vi "Autonomous Independent.vi"() -> ()   [LabVIEW 2014]
doc: "This VI is called when autonomous begins, and will automatically be terminated when autonomous ends. You can carry out timed or sensor driven robot movement independently without needing to return to the caller."
uses:
  <vilib>/Rock Robotics/WPI/Solenoid/WPI_SolenoidValue.ctl
  Robot Global Data.vi
  <vilib>/Rock Robotics/WPI/RobotDrive/WPI_RobotDriveGetSetRefNum.vi
  <vilib>/Rock Robotics/WPI/Solenoid/WPI_SolenoidSetEnum.vi
panel:
  out "One Ball Timer 1":u32
  out "Timer 2":u32
  out "Timer 1":u32
  out "Both Hands In":i32
  out "Av. Goalie 1 Ball Timer":u32
  out "Anti-Defense Iterations":dbl
  out "auton mode selected":string
  in  "pickup arm gripping speed":dbl=0.3
  in  "Speed Control":dbl=-0.46
  # "Be sure to right-click and choose Data Operations>>Make Current Value default if you want to save the array values with the VI"
  # "-0.46 < -0.48 <-0.51 -0.55< -0.43 < -0.5 < -0.58\n(Newest < New < Old < Oldest)"
  # "0.3"
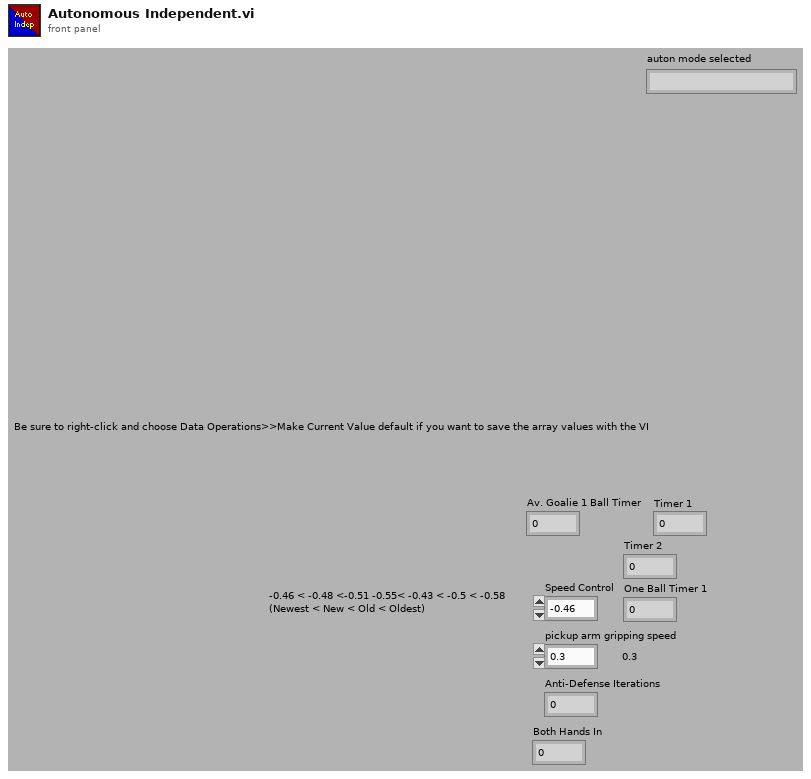
[diagram p1: front panel]
types:
  T1 = typedef "WPI_RobotDriveDevRef.ctl" = cluster{"DevStatus":errorcluster, "Motors[]":T2[], "Square Inputs":bool, "Max Output":dbl}
  T2 = typedef "WPI_MotorControlDeviceRef.ctl" = cluster{"DeviceStatus":errorcluster, "Type":enum16{"PWM", "CAN"}, "PWM":cluster{"Digital Module":T3, "PWM Channel":T4, "DeadBand":T5}, "CAN":cluster{"Device Number":u8, "Control Mode":T6, "Semaphore":T7, "Max Vout":dbl}, "Invert":bool, "TransformRef":T8, "InvTransformRef":T8}
  T3 = typedef "FPGA_TypedefDigitalModule.ctl" = enum16{"Digital Module 1", "Digital Module 2"}
  T4 = typedef "FPGA_DIOPWMChannel.ctl" = enum8{"PWM 1", "PWM 2", "PWM 3", "PWM 4", "PWM 5", "PWM 6", "PWM 7", "PWM 8", "PWM 9", "PWM 10", "Invalid"}
  T5 = typedef "WPI_PWMDeadband.ctl" = cluster{"Name":string, "maxPositivePwm":i32, "minPositivePwm":i32, "centerPwm":i32, "maxNegativePwm":i32, "minNegativePwm":i32, "angularRange":u16}
  T6 = typedef "WPI_CANJaguar_ControlMode.ctl" = enum8{"Percent VBus", "Current", "Speed", "Position", "Voltage"}
  T7 = typedef "Semaphore RefNum" = refnum<k1>
  T8 = typedef "WPI_PWMTransform_ConPane.ctl" = refnum<vi>
  T9 = typedef "WPI_AnalogChannelDevRef.ctl" = cluster{"DevStatus":errorcluster, "Analog Module":T10, "Analog Channel":T11}
  T10 = typedef "FPGA_TypedefAnalogModule.ctl" = enum16{"Analog Module 1", "Analog Module 2"}
  T11 = typedef "FPGA_AIChannel.ctl" = enum8{"AI 1", "AI 2", "AI 3", "AI 4", "AI 5", "AI 6", "AI 7", "AI 8", "Invalid"}
  T12 = typedef "WPI_SolenoidDevRef.ctl" = cluster{"DevStatus":errorcluster, "Solenoid Module":T13, "Forward Solenoid Channel":T14, "Reverse Solenoid Channel":T14}
  T13 = typedef "FPGA_TypedefSolenoidModule.ctl" = enum16{"Solenoid Module 1", "Solenoid Module 2"}
  T14 = typedef "WPI_SolenoidChannel.ctl" = enum8{"Solenoid 1", "Solenoid 2", "Solenoid 3", "Solenoid 4", "Solenoid 5", "Solenoid 6", "Solenoid 7", "Solenoid 8", "Invalid"}
  T15 = typedef "WPI_SolenoidValue.ctl" = enum16{"Off", "On", "Forward", "Reverse"}
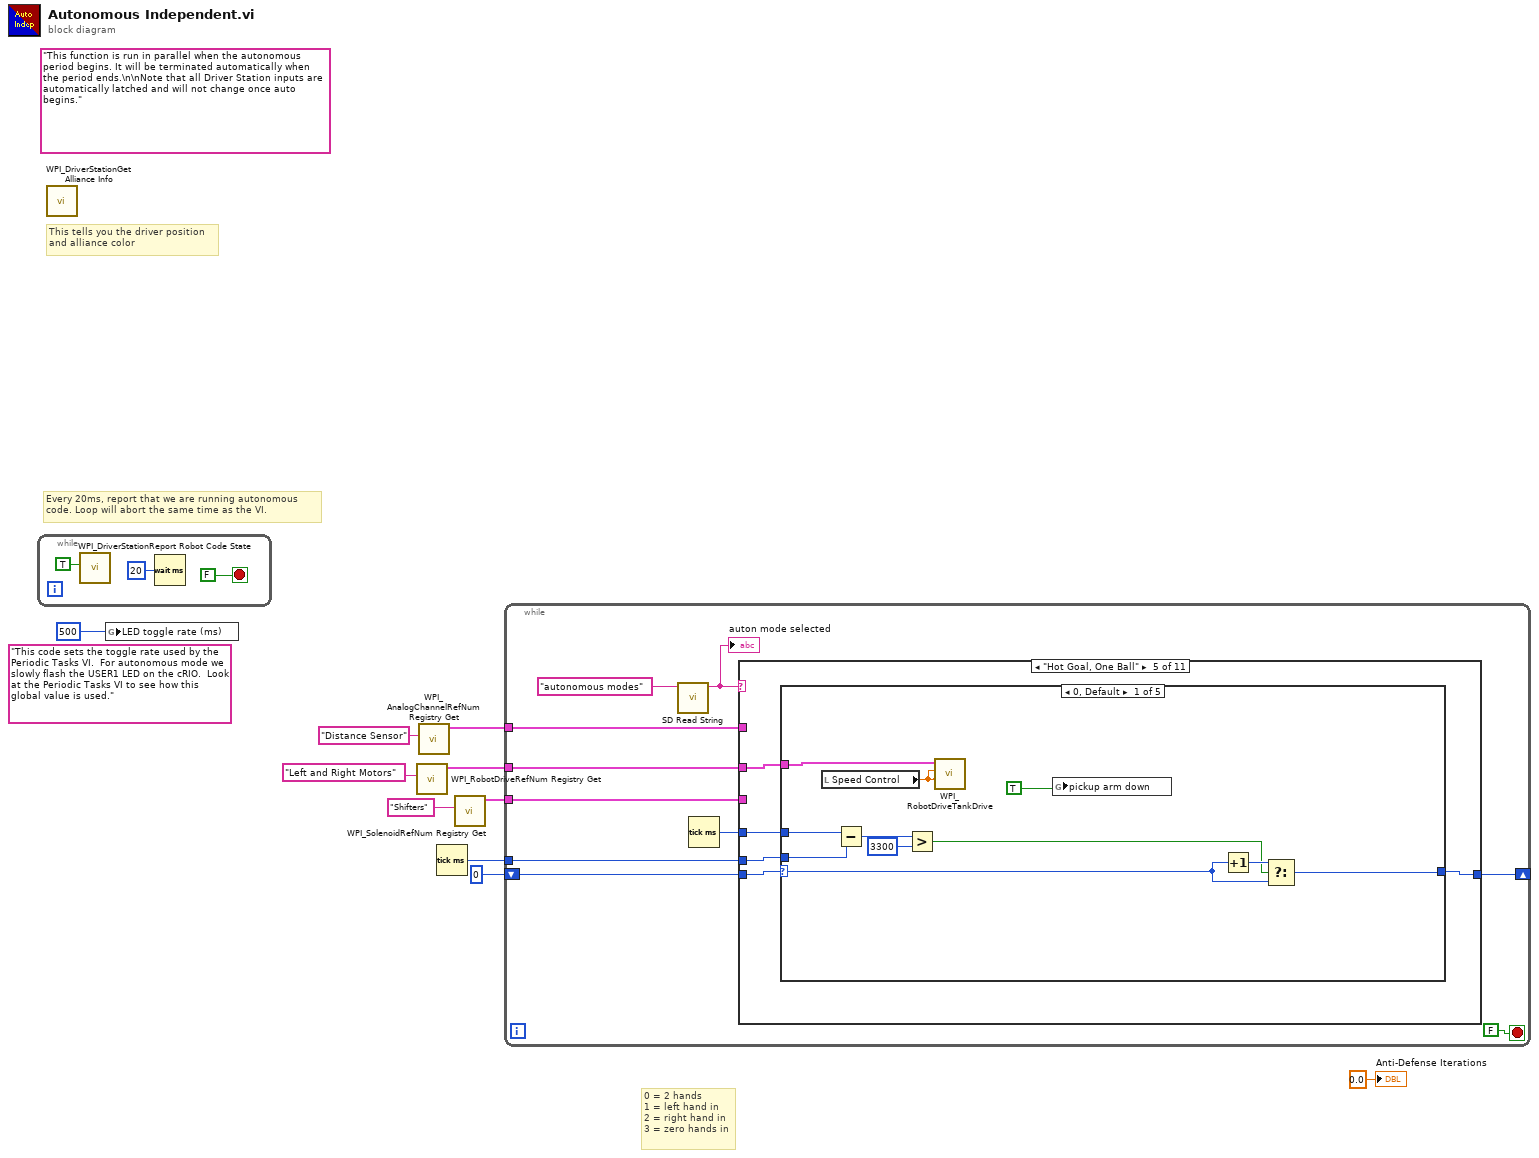
[diagram p0: block diagram]
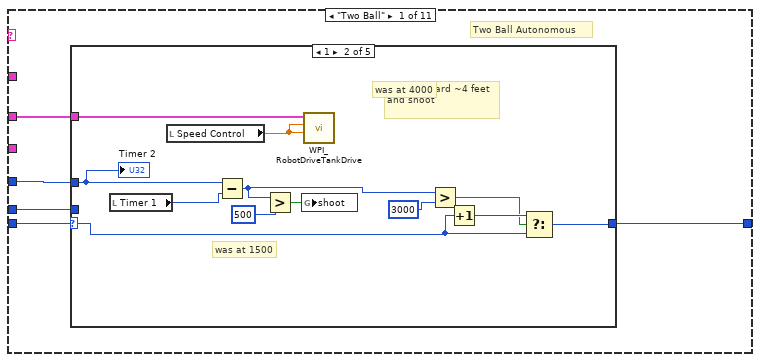
[diagram p2: hidden frame]
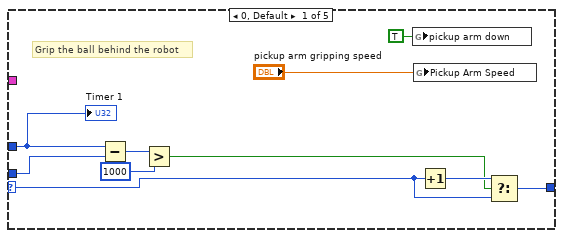
[diagram p3: hidden frame]
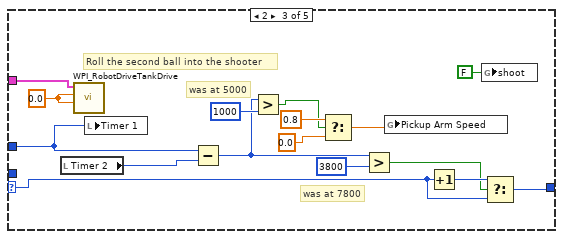
[diagram p4: hidden frame]
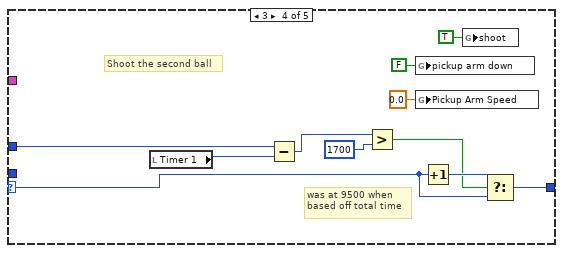
[diagram p5: hidden frame]
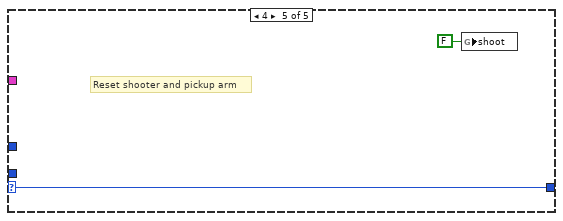
[diagram p6: hidden frame]
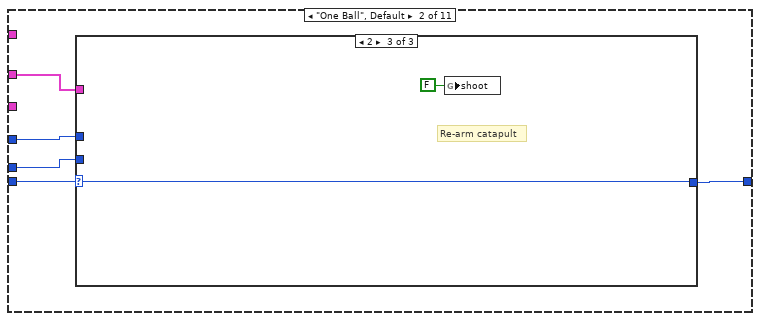
[diagram p7: hidden frame]
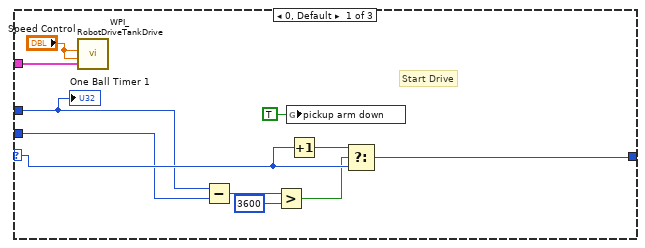
[diagram p8: hidden frame]
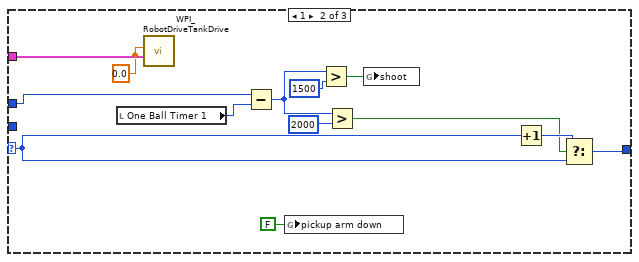
[diagram p9: hidden frame]
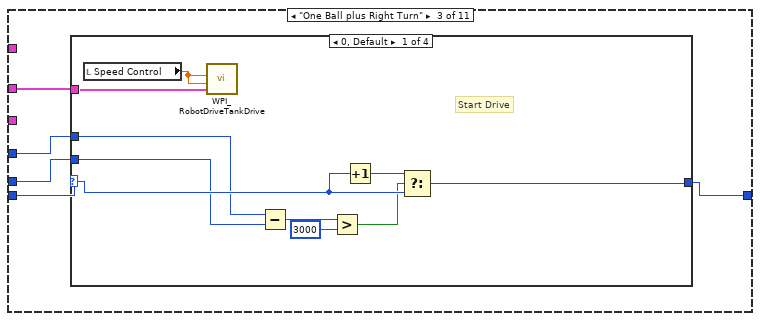
[diagram p10: hidden frame]
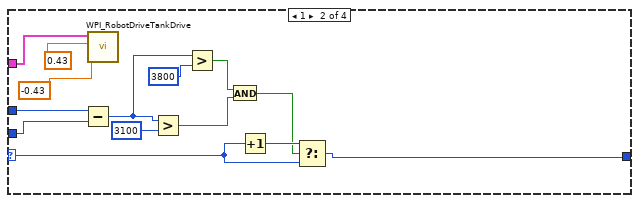
[diagram p11: hidden frame]
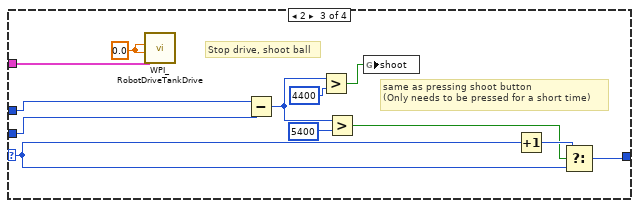
[diagram p12: hidden frame]
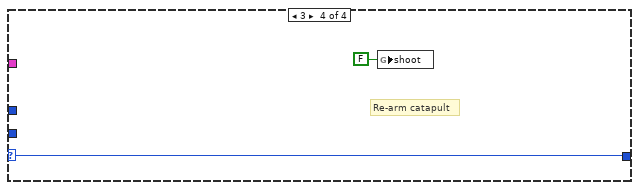
[diagram p13: hidden frame]
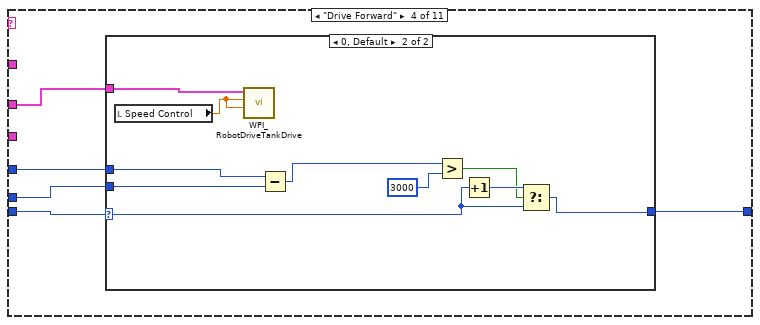
[diagram p14: hidden frame]
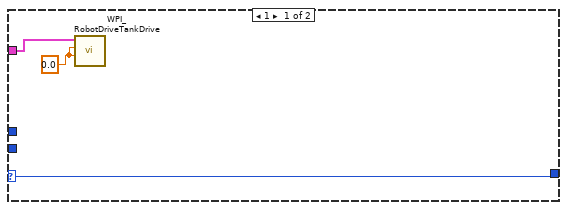
[diagram p15: hidden frame]
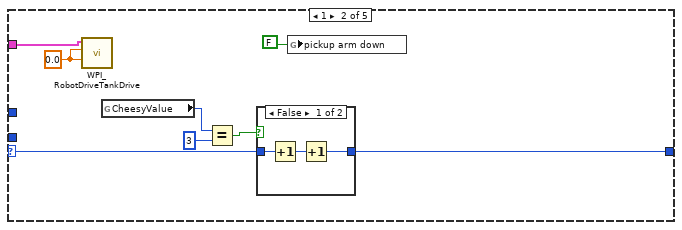
[diagram p16: hidden frame]
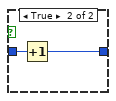
[diagram p17: hidden frame]
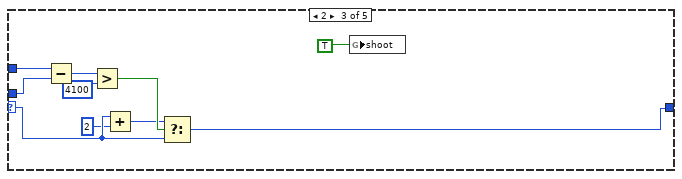
[diagram p18: hidden frame]
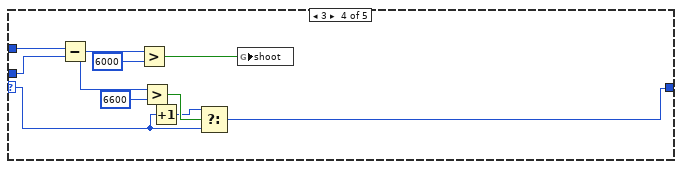
[diagram p19: hidden frame]
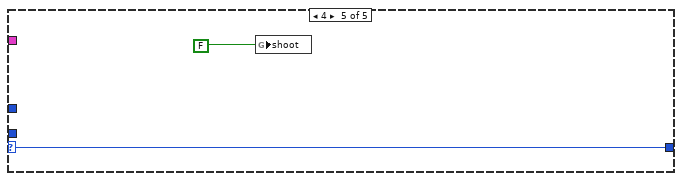
[diagram p20: hidden frame]
diagram:
  (unwired) "This code sets the toggle rate used by the Periodic Tasks VI.  For autonomous mode we slowly flash the USER1 LED on the cRIO.  Look at the Periodic Tasks VI to see how this global value is used."
  (unwired) "This function is run in parallel when the autonomous period begins. It will be terminated automatically when the period ends.\n\nNote that all Driver Station inputs are automatically latched and will not change once auto begins."
  # "0 = 2 hands\n1 = left hand in\n2 = right hand in\n3 = zero hands in"
  # "Every 20ms, report that we are running autonomous\ncode. Loop will abort the same time as the VI."
  # "This tells you the driver position\nand alliance color"
  n1 = while {
    stop <- FALSE stop-if-true
    n2 = call <vilib>:"WPI_DriverStationReport Robot Code State.vi"("Autonomous"=TRUE) -> ()  [unwired: 10 in, 1 out]
    n3 = Wait (ms)(milliseconds to wait=u32 20) -> ()  [unwired: 1 out]
  }
  n4 = call <vilib>:"WPI_DriverStationGet Alliance Info.vi"() -> ()  [unwired: 12 out]
  n5 = global write "Robot Global Data.vi" "LED toggle rate (ms)"(u32 500 ("LED ms toggle rate")) -> ()
  n6 = call <vilib>:"WPI_RobotDriveRefNum Registry Get.vi"("refnum name"="Left and Right Motors") -> ("RobotDriveDevRef"=w7:T1)  [unwired: 9 in, 1 out]
  n7 = call <vilib>:"WPI_AnalogChannelRefNum Registry Get.vi"("refnum name"="Distance Sensor") -> ("AIDeviceRef"=w1:T9)  [unwired: 9 in, 1 out]
  n8 = Tick Count (ms)() -> (millisecond timer value=w9:u32)
  n9 = call <vilib>:"WPI_SolenoidRefNum Registry Get.vi"("refnum name"="Shifters") -> ("SolenoidDevRef"=w4:T12)  [unwired: 9 in, 1 out]
  n10 = while {
    shift-right: [w19] -> _
    shift-left: 0 -> [w22]
    tunnel: w9 -> [w20]
    tunnel: w7 -> [w16]
    tunnel: w4 -> [w15]
    tunnel: w1 -> [w14]
    stop <- FALSE stop-if-true
    n11 = call <vilib>:"SD Read String.vi"("Name"="autonomous modes") -> ("String"=w17:string)  [unwired: 8 in, 2 out]
    "auton mode selected" <- w17
    n12 = Tick Count (ms)() -> (millisecond timer value=w21:u32)
    n13 = case shown="\"Hot Goal, One Ball\"" w17 {
      tunnel: w22 -> [w28 w83 w115 w155 w175 w227 w260 w308 w360 w472 w509]
      tunnel: w21 -> [w27 w82 w113 w157 w174 w223 w256 w307 w359 _ w508]
      tunnel: w20 -> [w26 w81 w114 w156 w173 _ _ w306 w358 _ w507]
      tunnel: [w25 w80 w111 w154 w176 w224 w257 w309 w357 w472 w506] -> w19
      tunnel: w16 -> [w24 w84 w112 w158 w172 w226 w259 w305 w361 w470 w505]
      tunnel: w15 -> [_ _ _ _ _ _ _ _ _ w469 _]
      tunnel: w14 -> [_ _ _ _ _ w228 w261 _ _ _ _]
      frame "Two Ball" {
        # "Two Ball Autonomous"
        n14 = case shown="1" w28 {
          selector: w28 -> [w30 w42 w65 w75 w79]
          tunnel: w27 -> [w29 w44 w52 w72 _]
          tunnel: w26 -> [w36 _ _ _ _]
          tunnel: [w33 w47 w62 w74 w79] -> w25
          tunnel: w24 -> [_ w50 w59 _ _]
          frame 0, Default {
            # "Grip the ball behind the robot"
            n15 = Subtract(x=w29, y=w36) -> (x-y=w35:u32)
            n16 = Greater?(x=w35, y=u32 1000) -> (0:w31:bool)
            n17 = global write "Robot Global Data.vi" "pickup arm down"(TRUE ("pickup arm down")) -> ()
            n18 = global write "Robot Global Data.vi" "Pickup Arm Speed"("pickup arm gripping speed") -> ()
            n19 = Increment(x=w30) -> (x+1=w32:u32)
            n20 = Select(t=w32, s=w31, f=w30) -> (s? t:f=w33:u32)
            "Timer 1" <- w29
          }
          frame 1 {
            # "was at 4000"
            # "was at 1500"
            # "Drive forward ~4 feet and shoot"
            n21 = local read "Timer 1"() -> (w39:u32)
            n22 = local read "Speed Control"() -> (w40:dbl)
            n23 = Subtract(x=w44, y=w39) -> (x-y=w46:u32)
            n24 = Greater?(x=w46, y=u32 500) -> (0:w41:bool)
            n25 = global write "Robot Global Data.vi" "shoot"(w41) -> ()
            n26 = call <vilib>:"WPI_RobotDriveTankDrive.vi"("Right axis value"=w40, "Left axis value"=w40, "RobotDriveDevRef"=w50) -> ()  [unwired: 6 in, 3 out]
            n27 = Greater?(x=w46, y=u32 3000) -> (0:w43:bool)
            n28 = Increment(x=w42) -> (x+1=w48:u32)
            n29 = Select(t=w48, s=w43, f=w42) -> (s? t:f=w47:u32)
            "Timer 2" <- w44
          }
          frame 2 {
            w60 = 0.0 ("Left axis value")
            # "was at 7800"
            # "was at 5000"
            # "Roll the second ball into the shooter"
            n30 = local read "Timer 2"() -> (w51:u32)
            n31 = call <vilib>:"WPI_RobotDriveTankDrive.vi"("Right axis value"=w60, "Left axis value"=w60, "RobotDriveDevRef"=w59) -> ()  [unwired: 6 in, 3 out]
            n32 = local write "Timer 1"(w52) -> ()
            n33 = Subtract(x=w52, y=w51) -> (x-y=w54:u32)
            n34 = Greater?(x=w54, y=u32 1000) -> (0:w53:bool)
            n35 = Select(t=0.8 ("Pickup Arm Speed"), s=w53, f=0.0) -> (s? t:f=w56:dbl)
            n36 = Greater?(x=w54, y=u32 3800) -> (0:w63:bool)
            n37 = global write "Robot Global Data.vi" "Pickup Arm Speed"(w56) -> ()
            n38 = Increment(x=w65) -> (x+1=w66:u32)
            n39 = global write "Robot Global Data.vi" "shoot"(FALSE ("shoot")) -> ()
            n40 = Select(t=w66, s=w63, f=w65) -> (s? t:f=w62:u32)
          }
          frame 3 {
            # "was at 9500 when\nbased off total time"
            # "Shoot the second ball"
            n41 = local read "Timer 1"() -> (w67:u32)
            n42 = Subtract(x=w72, y=w67) -> (x-y=w71:u32)
            n43 = Greater?(x=w71, y=u32 1700) -> (0:w69:bool)
            n44 = global write "Robot Global Data.vi" "pickup arm down"(FALSE ("pickup arm down")) -> ()
            n45 = global write "Robot Global Data.vi" "Pickup Arm Speed"(0.0 ("Pickup Arm Speed")) -> ()
            n46 = Increment(x=w75) -> (x+1=w76:u32)
            n47 = global write "Robot Global Data.vi" "shoot"(TRUE ("shoot")) -> ()
            n48 = Select(t=w76, s=w69, f=w75) -> (s? t:f=w74:u32)
          }
          frame 4 {
            # "Reset shooter and pickup arm"
            n49 = global write "Robot Global Data.vi" "shoot"(FALSE ("shoot")) -> ()
          }
        }
      }
      frame "One Ball", Default {
        n50 = case shown="2" w83 {
          selector: w83 -> [w93 w107 w110]
          tunnel: w84 -> [w95 w104 _]
          tunnel: w82 -> [w92 w102 _]
          tunnel: w81 -> [w91 _ _]
          tunnel: [w87 w105 w110] -> w80
          frame 0, Default {
            # "Start Drive"
            n51 = call <vilib>:"WPI_RobotDriveTankDrive.vi"("Right axis value"="Speed Control", "Left axis value"="Speed Control", "RobotDriveDevRef"=w95) -> ()  [unwired: 6 in, 3 out]
            n52 = Subtract(x=w92, y=w91) -> (x-y=w90:u32)
            n53 = Greater?(x=w90, y=u32 3600) -> (0:w88:bool)
            n54 = global write "Robot Global Data.vi" "pickup arm down"(TRUE ("pickup arm down")) -> ()
            n55 = Increment(x=w93) -> (x+1=w94:u32)
            n56 = Select(t=w94, s=w88, f=w93) -> (s? t:f=w87:u32)
            "One Ball Timer 1" <- w92
          }
          frame 1 {
            w103 = 0.0 ("Left axis value")
            n57 = local read "One Ball Timer 1"() -> (w96:u32)
            n58 = call <vilib>:"WPI_RobotDriveTankDrive.vi"("Right axis value"=w103, "Left axis value"=w103, "RobotDriveDevRef"=w104) -> ()  [unwired: 6 in, 3 out]
            n59 = Subtract(x=w102, y=w96) -> (x-y=w100:u32)
            n60 = global write "Robot Global Data.vi" "pickup arm down"(FALSE ("pickup arm down")) -> ()
            n61 = Greater?(x=w100, y=u32 1500) -> (0:w98:bool)
            n62 = Greater?(x=w100, y=u32 2000) -> (0:w101:bool)
            n63 = global write "Robot Global Data.vi" "shoot"(w98) -> ()
            n64 = Increment(x=w107) -> (x+1=w108:u32)
            n65 = Select(t=w108, s=w101, f=w107) -> (s? t:f=w105:u32)
          }
          frame 2 {
            # "Re-arm catapult"
            n66 = global write "Robot Global Data.vi" "shoot"(FALSE ("shoot")) -> ()
          }
        }
      }
      frame "One Ball plus Right Turn" {
        n67 = case shown="0, Default" w115 {
          selector: w115 -> [w123 w130 w150 w153]
          tunnel: w112 -> [w125 w134 w146 _]
          tunnel: w113 -> [w122 w139 w144 _]
          tunnel: w114 -> [w121 w138 w149 _]
          tunnel: [w117 w126 w147 w153] -> w111
          frame 0, Default {
            # "Start Drive"
            n68 = local read "Speed Control"() -> (w116:dbl)
            n69 = call <vilib>:"WPI_RobotDriveTankDrive.vi"("Right axis value"=w116, "Left axis value"=w116, "RobotDriveDevRef"=w125) -> ()  [unwired: 6 in, 3 out]
            n70 = Subtract(x=w122, y=w121) -> (x-y=w120:u32)
            n71 = Greater?(x=w120, y=u32 3000) -> (0:w118:bool)
            n72 = Increment(x=w123) -> (x+1=w124:u32)
            n73 = Select(t=w124, s=w118, f=w123) -> (s? t:f=w117:u32)
          }
          frame 1 {
            n74 = Subtract(x=w139, y=w138) -> (x-y=w136:u32)
            n75 = call <vilib>:"WPI_RobotDriveTankDrive.vi"("Right axis value"=-0.43, "Left axis value"=0.43, "RobotDriveDevRef"=w134) -> ()  [unwired: 6 in, 3 out]
            n76 = Greater?(x=w136, y=u32 3100) -> (0:w128:bool)
            n77 = Greater?(x=w136, y=u32 3800) -> (0:w129:bool)
            n78 = And(x=w129, y=w128) -> (x .and. y?=w127:bool)
            n79 = Increment(x=w130) -> (x+1=w131:u32)
            n80 = Select(t=w131, s=w127, f=w130) -> (s? t:f=w126:u32)
          }
          frame 2 {
            w145 = 0.0 ("Left axis value")
            # "same as pressing shoot button\n(Only needs to be pressed for a short time)"
            # "Stop drive, shoot ball"
            n81 = call <vilib>:"WPI_RobotDriveTankDrive.vi"("Right axis value"=w145, "Left axis value"=w145, "RobotDriveDevRef"=w146) -> ()  [unwired: 6 in, 3 out]
            n82 = Subtract(x=w144, y=w149) -> (x-y=w142:u32)
            n83 = Greater?(x=w142, y=u32 4400) -> (0:w140:bool)
            n84 = Greater?(x=w142, y=u32 5400) -> (0:w143:bool)
            n85 = global write "Robot Global Data.vi" "shoot"(w140) -> ()
            n86 = Increment(x=w150) -> (x+1=w151:u32)
            n87 = Select(t=w151, s=w143, f=w150) -> (s? t:f=w147:u32)
          }
          frame 3 {
            # "Re-arm catapult"
            n88 = global write "Robot Global Data.vi" "shoot"(FALSE ("shoot")) -> ()
          }
        }
      }
      frame "Drive Forward" {
        n89 = case shown="0, Default" w155 {
          selector: w155 -> [w159 w165]
          tunnel: w158 -> [w161 w169]
          tunnel: w157 -> [_ w171]
          tunnel: w156 -> [_ w170]
          tunnel: [w159 w164] -> w154
          frame 1 {
            w160 = 0.0 ("Right axis value")
            n90 = call <vilib>:"WPI_RobotDriveTankDrive.vi"("Right axis value"=w160, "Left axis value"=w160, "RobotDriveDevRef"=w161) -> ()  [unwired: 6 in, 3 out]
          }
          frame 0, Default {
            n91 = local read "Speed Control"() -> (w163:dbl)
            n92 = call <vilib>:"WPI_RobotDriveTankDrive.vi"("Right axis value"=w163, "Left axis value"=w163, "RobotDriveDevRef"=w169) -> ()  [unwired: 6 in, 3 out]
            n93 = Subtract(x=w171, y=w170) -> (x-y=w168:u32)
            n94 = Greater?(x=w168, y=u32 3000) -> (0:w162:bool)
            n95 = Increment(x=w165) -> (x+1=w166:u32)
            n96 = Select(t=w166, s=w162, f=w165) -> (s? t:f=w164:u32)
          }
        }
      }
      frame "Hot Goal, One Ball" {
        n97 = case shown="0, Default" w175 {
          selector: w175 -> [w186 w195 w205 w213 w221]
          tunnel: [w185 w194 w202 w212 w221] -> w176
          tunnel: w174 -> [w184 _ w210 w220 _]
          tunnel: w173 -> [w183 _ w209 w219 _]
          tunnel: w172 -> [w178 w193 _ _ _]
          frame 0, Default {
            n98 = local read "Speed Control"() -> (w179:dbl)
            n99 = Subtract(x=w184, y=w183) -> (x-y=w182:u32)
            n100 = Greater?(x=w182, y=u32 3300) -> (0:w180:bool)
            n101 = call <vilib>:"WPI_RobotDriveTankDrive.vi"("Right axis value"=w179, "Left axis value"=w179, "RobotDriveDevRef"=w178) -> ()  [unwired: 6 in, 3 out]
            n102 = global write "Robot Global Data.vi" "pickup arm down"(TRUE) -> ()
            n103 = Increment(x=w186) -> (x+1=w187:u32)
            n104 = Select(t=w187, s=w180, f=w186) -> (s? t:f=w185:u32)
          }
          frame 1 {
            w192 = 0.0 ("Left axis value")
            n105 = call <vilib>:"WPI_RobotDriveTankDrive.vi"("Right axis value"=w192, "Left axis value"=w192, "RobotDriveDevRef"=w193) -> ()  [unwired: 6 in, 3 out]
            n106 = global read "Robot Global Data.vi" "CheesyValue"() -> (w190:u8)
            n107 = Equal?(x=w190, y=u8 3) -> (x = y?=w191:bool)
            n108 = case shown="False" w191 {
              tunnel: w195 -> [w197 w200]
              tunnel: [w198 w199] -> w194
              frame False {
                n109 = Increment(x=w197) -> (x+1=w196:u32)
                n110 = Increment(x=w196) -> (x+1=w198:u32)
              }
              frame True {
                n111 = Increment(x=w200) -> (x+1=w199:u32)
              }
            }
            n112 = global write "Robot Global Data.vi" "pickup arm down"(FALSE) -> ()
          }
          frame 2 {
            n113 = Subtract(x=w210, y=w209) -> (x-y=w208:u32)
            n114 = Greater?(x=w208, y=u32 4100) -> (0:w206:bool)
            n115 = Add(x=w205, y=2) -> (x+y=w203:u32)
            n116 = Select(t=w203, s=w206, f=w205) -> (s? t:f=w202:u32)
            n117 = global write "Robot Global Data.vi" "shoot"(TRUE) -> ()
          }
          frame 3 {
            n118 = Subtract(x=w220, y=w219) -> (x-y=w217:u32)
            n119 = Greater?(x=w217, y=u32 6000) -> (0:w211:bool)
            n120 = Greater?(x=w217, y=u32 6600) -> (0:w215:bool)
            n121 = Increment(x=w213) -> (x+1=w214:u32)
            n122 = Select(t=w214, s=w215, f=w213) -> (s? t:f=w212:u32)
            n123 = global write "Robot Global Data.vi" "shoot"(w211) -> ()
          }
          frame 4 {
            n124 = global write "Robot Global Data.vi" "shoot"(FALSE) -> ()
          }
        }
      }
      frame "Sensorjxsthrxht" {
        n125 = call <vilib>:"WPI_AnalogChannelGetVoltage.vi"("AIDeviceRef"=w228) -> ("Voltage"=w225:dbl)  [unwired: 8 in, 2 out]
        n126 = case shown="0, Default" w227 {
          selector: w227 -> [_ _ w255]
          tunnel: w226 -> [w241 w253 _]
          tunnel: w225 -> [w233 _ _]
          tunnel: [w236 w243 w255] -> w224
          tunnel: w223 -> [w235 w250 _]
          frame 0, Default {
            n127 = local read "Speed Control"() -> (w231:dbl)
            n128 = local write "Timer 1"(w235) -> ()
            n129 = Subtract(x=w231, y=0.015) -> (x-y=w230:dbl)
            n130 = call <vilib>:"WPI_RobotDriveTankDrive.vi"("Right axis value"=w230, "Left axis value"=w231, "RobotDriveDevRef"=w241) -> ()  [unwired: 6 in, 3 out]
            n131 = global write "Robot Global Data.vi" "pickup arm down"(TRUE ("pickup arm down")) -> ()
            n132 = Less?(x=w233, y=1.7) -> (x < y?=w239:bool)
            n133 = call <vilib>:"SD Write Number.vi"("Numeric"=w233, "Name"="Distance Sensor Voltage") -> ()  [unwired: 8 in, 2 out]
            n134 = Select(t=1, s=w239, f=0) -> (s? t:f=w236:i32)
          }
          frame 1 {
            w252 = 0.0 ("Left axis value")
            n135 = local read "Timer 1"() -> (w249:u32)
            n136 = call <vilib>:"WPI_RobotDriveTankDrive.vi"("Right axis value"=w252, "Left axis value"=w252, "RobotDriveDevRef"=w253) -> ()  [unwired: 6 in, 3 out]
            n137 = Subtract(x=w250, y=w249) -> (x-y=w248:u32)
            n138 = Greater?(x=w248, y=u32 1000) -> (0:w246:bool)
            n139 = global write "Robot Global Data.vi" "pickup arm down"(FALSE ("pickup arm down")) -> ()
            n140 = global write "Robot Global Data.vi" "shoot"(TRUE ("shoot")) -> ()
            n141 = Select(t=u32 2 ("y"), s=w246, f=u32 1 ("y")) -> (s? t:f=w243:u32)
          }
          frame 2 {
            n142 = global write "Robot Global Data.vi" "shoot"(FALSE ("shoot")) -> ()
          }
        }
      }
      frame "Two Ball Sensor" {
        n143 = call <vilib>:"WPI_AnalogChannelGetVoltage.vi"("AIDeviceRef"=w261) -> ("Voltage"=w258:dbl)  [unwired: 8 in, 2 out]
        n144 = case shown="0, Default" w260 {
          selector: w260 -> [_ _ _ w297]
          tunnel: w259 -> [w275 w287 _ _]
          tunnel: w258 -> [w267 _ _ _]
          tunnel: [w270 w281 w291 w297] -> w257
          tunnel: w256 -> [w269 w276 w288 w302]
          frame 0, Default {
            n145 = local read "pickup arm gripping speed"() -> (w262:dbl)
            n146 = local read "Speed Control"() -> (w265:dbl)
            n147 = local write "Timer 1"(w269) -> ()
            n148 = Subtract(x=w265, y=0.015) -> (x-y=w264:dbl)
            n149 = call <vilib>:"WPI_RobotDriveTankDrive.vi"("Right axis value"=w264, "Left axis value"=w265, "RobotDriveDevRef"=w275) -> ()  [unwired: 6 in, 3 out]
            n150 = global write "Robot Global Data.vi" "pickup arm down"(TRUE ("pickup arm down")) -> ()
            n151 = global write "Robot Global Data.vi" "Pickup Arm Speed"(w262) -> ()
            n152 = Less?(x=w267, y=1.75) -> (x < y?=w273:bool)
            n153 = call <vilib>:"SD Write Number.vi"("Numeric"=w267, "Name"="Distance Sensor Voltage") -> ()  [unwired: 8 in, 2 out]
            n154 = Select(t=1, s=w273, f=0) -> (s? t:f=w270:i32)
          }
          frame 1 {
            w286 = 0.0 ("Left axis value")
            n155 = local read "Timer 1"() -> (w285:u32)
            n156 = call <vilib>:"WPI_RobotDriveTankDrive.vi"("Right axis value"=w286, "Left axis value"=w286, "RobotDriveDevRef"=w287) -> ()  [unwired: 6 in, 3 out]
            n157 = local write "Timer 2"(w276) -> ()
            n158 = Subtract(x=w276, y=w285) -> (x-y=w279:u32)
            n159 = Less?(x=w279, y=u32 1000) -> (x < y?=w280:bool)
            n160 = global write "Robot Global Data.vi" "shoot"(w280) -> ()
            n161 = Greater?(x=w279, y=u32 2000) -> (0:w277:bool)
            n162 = Select(t=u32 2 ("y"), s=w277, f=u32 1 ("y")) -> (s? t:f=w281:u32)
          }
          frame 2 {
            n163 = local read "Timer 2"() -> (w295:u32)
            n164 = local write "Timer 1"(w288) -> ()
            n165 = Subtract(x=w288, y=w295) -> (x-y=w294:u32)
            n166 = Greater?(x=w294, y=u32 2500) -> (0:w289:bool)
            n167 = global write "Robot Global Data.vi" "Pickup Arm Speed"(1.0 ("Pickup Arm Speed")) -> ()
            n168 = Select(t=u32 3 ("y"), s=w289, f=u32 2 ("y")) -> (s? t:f=w291:u32)
          }
          frame 3 {
            n169 = local read "Timer 1"() -> (w301:u32)
            n170 = Subtract(x=w302, y=w301) -> (x-y=w300:u32)
            n171 = Less?(x=w300, y=u32 1000) -> (x < y?=w298:bool)
            n172 = global write "Robot Global Data.vi" "shoot"(w298) -> ()
            n173 = global write "Robot Global Data.vi" "pickup arm down"(FALSE ("pickup arm down")) -> ()
            n174 = global write "Robot Global Data.vi" "Pickup Arm Speed"(0.0 ("Pickup Arm Speed")) -> ()
          }
        }
      }
      frame "Avoid Goalie one Ball" {
        n175 = case shown="1" w308 {
          selector: w308 -> [w319 _ w347 w355]
          tunnel: [w318 w321 w349 w355] -> w309
          tunnel: w307 -> [w317 w328 w354 _]
          tunnel: w306 -> [w316 _ _ _]
          tunnel: w305 -> [w311 w331 _ _]
          frame 0, Default {
            n176 = local read "Speed Control"() -> (w312:dbl)
            n177 = Subtract(x=w317, y=w316) -> (x-y=w315:u32)
            n178 = Greater?(x=w315, y=u32 2500) -> (0:w313:bool)
            n179 = call <vilib>:"WPI_RobotDriveTankDrive.vi"("Right axis value"=w312, "Left axis value"=w312, "RobotDriveDevRef"=w311) -> ()  [unwired: 6 in, 3 out]
            n180 = global write "Robot Global Data.vi" "pickup arm down"(TRUE) -> ()
            n181 = Increment(x=w319) -> (x+1=w320:u32)
            n182 = Select(t=w320, s=w313, f=w319) -> (s? t:f=w318:u32)
          }
          frame 1 {
            n183 = global read "Robot Global Data.vi" "CheesyValue"() -> (w332:u8)
            n184 = case shown="0" w332 {
              tunnel: [0.0 ("Left axis value") -0.3 ("Left axis value") 0.3 ("Left axis value") 0.0 ("Left axis value")] -> w330
              tunnel: [0.0 ("Left axis value") 0.3 ("Left axis value") -0.3 ("Left axis value") 0.0 ("Left axis value")] -> w329
              tunnel: [w333 0 0 0] -> w326
              frame 0 {
                n185 = local read "Both Hands In"() -> (w334:i32)
                n186 = Increment(x=w334) -> (x+1=w333:i32)
              }
              frame 1 {
              }
              frame 2 {
              }
              frame 3, Default {
              }
            }
            "Both Hands In" <- w326
            n187 = global write "Robot Global Data.vi" "pickup arm down"(FALSE) -> ()
            n188 = call <vilib>:"WPI_RobotDriveTankDrive.vi"("Right axis value"=w329, "Left axis value"=w330, "RobotDriveDevRef"=w331) -> ()  [unwired: 6 in, 3 out]
            n189 = Greater?(x=w326, y=20) -> (0:w322:bool)
            n190 = Select(t=2, s=w322, f=1) -> (s? t:f=w321:i32)
            "Av. Goalie 1 Ball Timer" <- w328
          }
          frame 2 {
            n191 = local read "Av. Goalie 1 Ball Timer"() -> (w346:u32)
            n192 = Subtract(x=w354, y=w346) -> (x-y=w353:u32)
            n193 = Increment(x=w347) -> (x+1=w350:u32)
            n194 = Greater?(x=w353, y=u32 1200) -> (0:w351:bool)
            n195 = Select(t=w350, s=w351, f=w347) -> (s? t:f=w349:u32)
            n196 = global write "Robot Global Data.vi" "shoot"(TRUE) -> ()
          }
          frame 3 {
            n197 = global write "Robot Global Data.vi" "shoot"(FALSE) -> ()
          }
        }
      }
      frame "Hot Goal, Two Ball" {
        n198 = case shown="0, Default" w360 {
          selector: w360 -> [w364 w373 w386 w398 w408 w423 w437 w454 w462]
          tunnel: w361 -> [_ w376 w384 w396 w411 w416 w444 w451 _]
          tunnel: w359 -> [w366 w375 _ w403 w410 w429 w442 w460 _]
          tunnel: w358 -> [w365 w374 _ w402 w409 w428 w441 w459 _]
          tunnel: [w363 w372 w385 w397 w407 w422 w436 w452 w462] -> w357
          frame 0, Default {
            n199 = Subtract(x=w366, y=w365) -> (x-y=w370:u32)
            n200 = Greater?(x=w370, y=u32 1000) -> (0:w367:bool)
            n201 = global write "Robot Global Data.vi" "pickup arm down"(TRUE ("pickup arm down")) -> ()
            n202 = global write "Robot Global Data.vi" "Pickup Arm Speed"(0.3 ("Pickup Arm Speed")) -> ()
            n203 = Increment(x=w364) -> (x+1=w368:u32)
            n204 = Select(t=w368, s=w367, f=w364) -> (s? t:f=w363:u32)
          }
          frame 1 {
            # "Drive forward ~4 feet and shoot"
            n205 = local read "Speed Control"() -> (w381:dbl)
            n206 = Subtract(x=w375, y=w374) -> (x-y=w379:u32)
            n207 = call <vilib>:"WPI_RobotDriveTankDrive.vi"("Right axis value"=w381, "Left axis value"=w381, "RobotDriveDevRef"=w376) -> ()  [unwired: 6 in, 3 out]
            n208 = Greater?(x=w379, y=u32 3000) -> (0:w377:bool)
            n209 = Increment(x=w373) -> (x+1=w380:u32)
            n210 = Select(t=w380, s=w377, f=w373) -> (s? t:f=w372:u32)
          }
          frame 2 {
            w383 = 0.0 ("Left axis value")
            n211 = call <vilib>:"WPI_RobotDriveTankDrive.vi"("Right axis value"=w383, "Left axis value"=w383, "RobotDriveDevRef"=w384) -> ()  [unwired: 6 in, 3 out]
            n212 = global read "Robot Global Data.vi" "Hot Indicator"() -> (w382:bool)
            n213 = case shown="True" w382 {
              tunnel: w386 -> [w388 w391]
              tunnel: [w387 w389] -> w385
              frame False {
                n214 = Increment(x=w388) -> (x+1=w387:u32)
              }
              frame True {
                n215 = Increment(x=w391) -> (x+1=w390:u32)
                n216 = Increment(x=w390) -> (x+1=w389:u32)
              }
            }
          }
          frame 3 {
            n217 = local read "Speed Control"() -> (w392:dbl)
            n218 = Subtract(x=w403, y=w402) -> (x-y=w401:u32)
            n219 = Greater?(x=w401, y=u32 3500) -> (0:w399:bool)
            n220 = Negate(x=w392) -> (-x=w393:dbl)
            n221 = Increment(x=w398) -> (x+1=w395:u32)
            n222 = call <vilib>:"WPI_RobotDriveTankDrive.vi"("Right axis value"=w393, "Left axis value"=w392, "RobotDriveDevRef"=w396) -> ()  [unwired: 6 in, 3 out]
            n223 = Increment(x=w395) -> (x+1=w394:u32)
            n224 = Select(t=w394, s=w399, f=w398) -> (s? t:f=w397:u32)
          }
          frame 4 {
            n225 = local read "Speed Control"() -> (w405:dbl)
            n226 = Subtract(x=w410, y=w409) -> (x-y=w414:u32)
            n227 = Greater?(x=w414, y=u32 3500) -> (0:w412:bool)
            n228 = Negate(x=w405) -> (-x=w404:dbl)
            n229 = Increment(x=w408) -> (x+1=w406:u32)
            n230 = call <vilib>:"WPI_RobotDriveTankDrive.vi"("Right axis value"=w405, "Left axis value"=w404, "RobotDriveDevRef"=w411) -> ()  [unwired: 6 in, 3 out]
            n231 = Select(t=w406, s=w412, f=w408) -> (s? t:f=w407:u32)
          }
          frame 5 {
            w415 = 0.0 ("Left axis value")
            n232 = call <vilib>:"WPI_RobotDriveTankDrive.vi"("Right axis value"=w415, "Left axis value"=w415, "RobotDriveDevRef"=w416) -> ()  [unwired: 6 in, 3 out]
            n233 = Subtract(x=w429, y=w428) -> (x-y=w419:u32)
            n234 = Greater?(x=w419, y=u32 4000) -> (0:w421:bool)
            n235 = Greater?(x=w419, y=u32 7000) -> (0:w425:bool)
            n236 = Less?(x=w419, y=u32 4500) -> (x < y?=w420:bool)
            n237 = And(x=w421, y=w420) -> (x .and. y?=w417:bool)
            n238 = Increment(x=w423) -> (x+1=w424:u32)
            n239 = Select(t=w424, s=w425, f=w423) -> (s? t:f=w422:u32)
            n240 = global write "Robot Global Data.vi" "shoot"(w417) -> ()
          }
          frame 6 {
            n241 = local read "Speed Control"() -> (w443:dbl)
            n242 = global read "Robot Global Data.vi" "Hot Indicator"() -> (w430:bool)
            n243 = Subtract(x=w442, y=w441) -> (x-y=w433:u32)
            n244 = case shown="True" w430 {
              tunnel: w443 -> [w446 w448]
              tunnel: [w446 w449] -> w434
              tunnel: [w447 w448] -> w435
              frame False {
                n245 = Negate(x=w446) -> (-x=w447:dbl)
              }
              frame True {
                n246 = Negate(x=w448) -> (-x=w449:dbl)
              }
            }
            n247 = Less?(x=w433, y=u32 7500) -> (x < y?=w431:bool)
            n248 = call <vilib>:"WPI_RobotDriveTankDrive.vi"("Right axis value"=w434, "Left axis value"=w435, "RobotDriveDevRef"=w444) -> ()  [unwired: 6 in, 3 out]
            n249 = global write "Robot Global Data.vi" "pickup arm down"(w431) -> ()
            n250 = Greater?(x=w433, y=u32 7900) -> (0:w439:bool)
            n251 = Increment(x=w437) -> (x+1=w438:u32)
            n252 = Select(t=w438, s=w439, f=w437) -> (s? t:f=w436:u32)
            n253 = global write "Robot Global Data.vi" "Pickup Arm Speed"(0.8 ("Pickup Arm Speed")) -> ()
          }
          frame 7 {
            w450 = 0.0 ("Left axis value")
            n254 = Subtract(x=w460, y=w459) -> (x-y=w458:u32)
            n255 = call <vilib>:"WPI_RobotDriveTankDrive.vi"("Right axis value"=w450, "Left axis value"=w450, "RobotDriveDevRef"=w451) -> ()  [unwired: 6 in, 3 out]
            n256 = Greater?(x=w458, y=u32 8900) -> (0:w455:bool)
            n257 = Increment(x=w454) -> (x+1=w453:u32)
            n258 = Select(t=w453, s=w455, f=w454) -> (s? t:f=w452:u32)
            n259 = global write "Robot Global Data.vi" "shoot"(TRUE) -> ()
            n260 = global write "Robot Global Data.vi" "Pickup Arm Speed"(0.0 ("Pickup Arm Speed")) -> ()
          }
          frame 8 {
            n261 = global write "Robot Global Data.vi" "shoot"(FALSE ("shoot")) -> ()
          }
        }
      }
      frame "Anti Defense" {
        n262 = local read "Anti-Defense Iterations"() -> (w465:dbl)
        n263 = global read "Robot Global Data.vi" "CheesyValue"() -> (w471:u8)
        n264 = case shown="0, Default" w471 {
          tunnel: w470 -> [w479 w492 w498 w503]
          tunnel: w469 -> [w481 w491 w497 w502]
          tunnel: [w481 w491 w497 w502] -> w468
          tunnel: [WPI_SolenoidValue."On" ("Value") WPI_SolenoidValue."Off" ("Value") WPI_SolenoidValue."Off" ("Value") WPI_SolenoidValue."Off" ("Value")] -> w467
          tunnel: w465 -> [w477 w488 w494 w500]
          tunnel: [w477 w489 w495 w500] -> w464
          frame 0, Default {
            n265 = Greater?(x=w477, y=0.0) -> (0:w475:bool)
            n266 = case shown="True" w475 {
              tunnel: w479 -> [w484 w487]
              tunnel: [w484 w487] -> w478
              tunnel: [0.4 -0.4 ("Right axis value")] -> w474
              tunnel: [-0.4 0.4 ("Right axis value")] -> w473
              frame False {
              }
              frame True {
              }
            }
            n267 = call <vilib>:"WPI_RobotDriveTankDrive.vi"("Right axis value"=w473, "Left axis value"=w474, "RobotDriveDevRef"=w478) -> ()  [unwired: 6 in, 3 out]
          }
          frame 1 {
            w493 = 0.4 ("Right axis value")
            n268 = call <vilib>:"WPI_RobotDriveTankDrive.vi"("Right axis value"=w493, "Left axis value"=w493, "RobotDriveDevRef"=w492) -> ()  [unwired: 6 in, 3 out]
            n269 = Increment(x=w488) -> (x+1=w489:dbl)
          }
          frame 2 {
            w499 = -0.4 ("Right axis value")
            n270 = call <vilib>:"WPI_RobotDriveTankDrive.vi"("Right axis value"=w499, "Left axis value"=w499, "RobotDriveDevRef"=w498) -> ()  [unwired: 6 in, 3 out]
            n271 = Decrement(x=w494) -> (x-1=w495:dbl)
          }
          frame 3 {
            w504 = 0.0 ("Right axis value")
            n272 = call <vilib>:"WPI_RobotDriveTankDrive.vi"("Right axis value"=w504, "Left axis value"=w504, "RobotDriveDevRef"=w503) -> ()  [unwired: 6 in, 3 out]
          }
        }
        n273 = local write "Anti-Defense Iterations"(w464) -> ()
        n274 = call-poly <vilib>:"WPI_SolenoidSet.vi"("Value"=w467, "SolenoidDevRef"=w468) -> ()  [unwired: 8 in, 2 out]
        n275 = global write "Robot Global Data.vi" "Pickup Arm Speed"(0.0) -> ()
      }
      frame "Test" {
        # "Two Ball Autonomous- Shoot FIRST"
        n276 = case shown="0, Default" w509 {
          selector: w509 -> [w518 w528 w537 w546]
          tunnel: w508 -> [w510 w521 w543 _]
          tunnel: w507 -> [w517 w522 w533 _]
          tunnel: [w514 w527 w536 w546] -> w506
          tunnel: w505 -> [_ _ w545 w549]
          frame 0, Default {
            # "Shoot the first ball"
            n277 = Subtract(x=w510, y=w517) -> (x-y=w516:u32)
            n278 = Greater?(x=w516, y=u32 100) -> (0:w512:bool)
            n279 = global read "Robot Global Data.vi" "Catapult Switch Triggered"() -> (w513:bool)
            n280 = Increment(x=w518) -> (x+1=w519:u32)
            n281 = And(x=w513, y=w512) -> (x .and. y?=w511:bool)
            n282 = global write "Robot Global Data.vi" "shoot"(TRUE ("shoot")) -> ()
            n283 = Select(t=w519, s=w511, f=w518) -> (s? t:f=w514:u32)
          }
          frame 1 {
            # "Wait for shooter to reset"
            n284 = Subtract(x=w521, y=w522) -> (x-y=w525:u32)
            n285 = Greater?(x=w525, y=u32 500) -> (0:w523:bool)
            n286 = Greater?(x=w525, y=u32 3500) -> (0:w530:bool)
            n287 = global write "Robot Global Data.vi" "pickup arm down"(w523) -> ()
            n288 = global write "Robot Global Data.vi" "Pickup Arm Speed"(1.0 ("Pickup Arm Speed")) -> ()
            n289 = Increment(x=w528) -> (x+1=w529:u32)
            n290 = Select(t=w529, s=w530, f=w528) -> (s? t:f=w527:u32)
            n291 = global write "Robot Global Data.vi" "shoot"(FALSE ("shoot")) -> ()
          }
          frame 2 {
            # "Drive forward ~4 feet and shoot"
            n292 = local read "Speed Control"() -> (w544:dbl)
            n293 = call <vilib>:"WPI_RobotDriveTankDrive.vi"("Right axis value"=w544, "Left axis value"=w544, "RobotDriveDevRef"=w545) -> ()  [unwired: 6 in, 3 out]
            n294 = Subtract(x=w543, y=w533) -> (x-y=w535:u32)
            n295 = Greater?(x=w535, y=u32 2500) -> (0:w541:bool)
            n296 = global write "Robot Global Data.vi" "shoot"(w541) -> ()
            n297 = Greater?(x=w535, y=u32 2800) -> (0:w539:bool)
            n298 = Increment(x=w537) -> (x+1=w538:u32)
            n299 = global write "Robot Global Data.vi" "pickup arm down"(FALSE ("pickup arm down")) -> ()
            n300 = Select(t=w538, s=w539, f=w537) -> (s? t:f=w536:u32)
          }
          frame 3 {
            w548 = 0.0 ("Left axis value")
            # "Allow the shooter to reset"
            n301 = call <vilib>:"WPI_RobotDriveTankDrive.vi"("Right axis value"=w548, "Left axis value"=w548, "RobotDriveDevRef"=w549) -> ()  [unwired: 6 in, 3 out]
            n302 = global write "Robot Global Data.vi" "shoot"(FALSE ("shoot")) -> ()
          }
        }
      }
    }
  }
  "Anti-Defense Iterations" <- 0.0 ("Anti-Defense Iterations")
